vi "IB_RW_Convert_Path_to_Relative.vi"(8 "error in (no error)":errorcluster, 10 "commonPath":path, 11 "absolutePath":path) -> (0 "error out":errorcluster, 2 "relativeType":T1, 3 "newPath":path)   [LabVIEW 2020]
uses:
  <vilib>/AppBuilder/AB_Relative_Path_Type.ctl
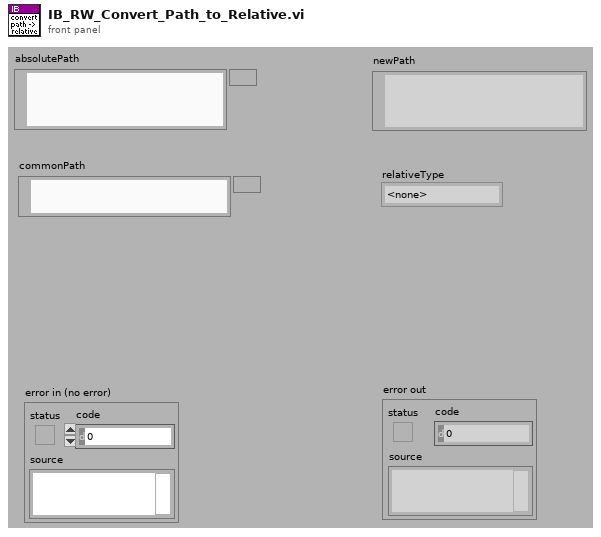
[diagram p1: front panel]
types:
  T1 = typedef "AB_Relative_Path_Type.ctl" = enum16{"<none>", "relativeToCommon", "relativeToAppDir", "relativeToProject"}
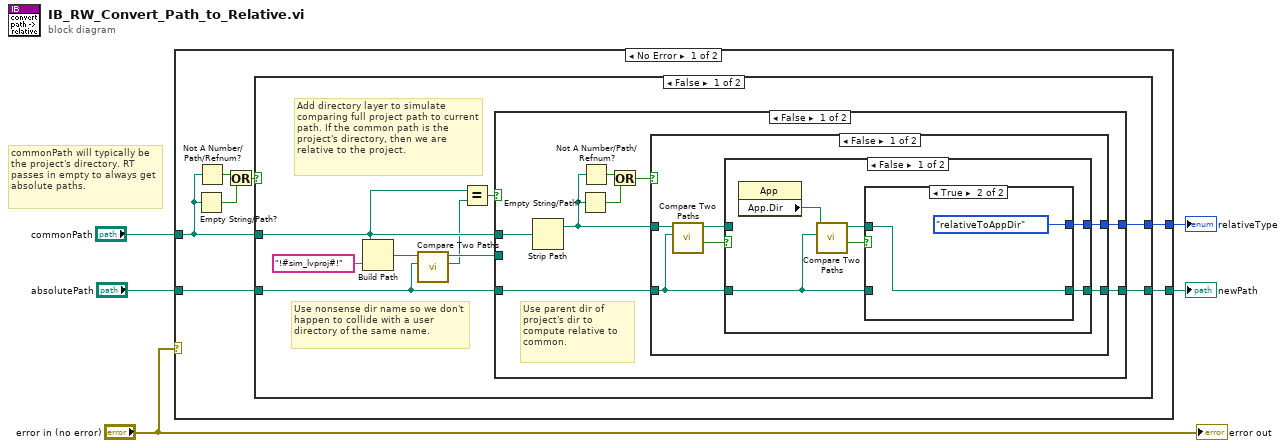
[diagram p0: block diagram]
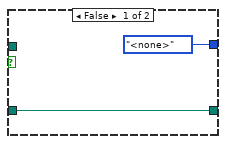
[diagram p2: hidden frame]
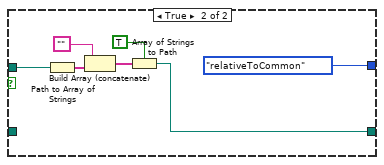
[diagram p3: hidden frame]
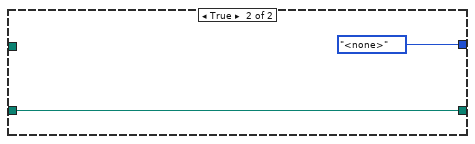
[diagram p4: hidden frame]
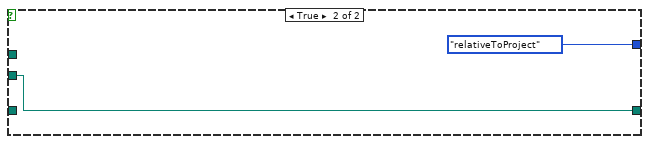
[diagram p5: hidden frame]
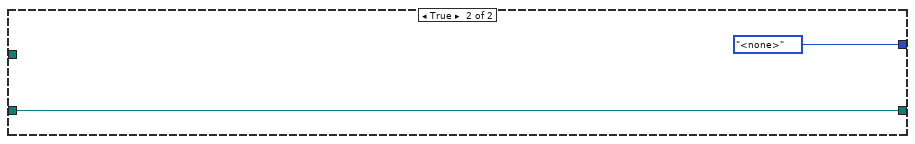
[diagram p6: hidden frame]
diagram:
  # "commonPath will typically be the project's directory. RT passes in empty to always get absolute paths."
  n1 = case shown="No Error" "error in (no error)" {
    tunnel: "commonPath" -> [w7 _]
    tunnel: "absolutePath" -> [w12 w59]
    tunnel: [w11 w59] -> w3
    tunnel: [w10 _] -> w2
    frame No Error {
      n2 = Empty String/Path?(string/path=w7) -> (empty?=w9:bool)
      n3 = Not A Number/Path/Refnum?(number/path/refnum=w7) -> (NaN/Path/Refnum?=w8:bool)
      n4 = Or(x=w8, y=w9) -> (x .or. y?=w6:bool)
      n5 = case shown="False" w6 {
        tunnel: w12 -> [w16 w58]
        tunnel: [w21 w58] -> w11
        tunnel: [w20 AB_Relative_Path_Type."<none>" ("relativeType")] -> w10
        tunnel: w7 -> [w15 _]
        frame False {
          # "Use nonsense dir name so we don't happen to collide with a user directory of the same name."
          # "Add directory layer to simulate comparing full project path to current path. If the common path is the project's directory, then we are relative to the project."
          n6 = Build Path(base path=w15, name or relative path="!#sim_lvproj#!") -> (appended path=w17:path)
          n7 = call <vilib>:"Compare Two Paths.vi"("Path 2"=w16, "Path 1"=w17) -> ("Common Path"=w14:path, "Relative Path from 1 to 2"=w18:path)  [unwired: 6 in, 2 out]
          n8 = Equal?(x=w15, y=w14) -> (x = y?=w13:bool)
          n9 = case shown="False" w13 {
            tunnel: [w29 w56] -> w21
            tunnel: [w28 AB_Relative_Path_Type."relativeToProject" ("relativeType")] -> w20
            tunnel: w15 -> [w23 _]
            tunnel: w16 -> [w22 _]
            tunnel: w18 -> [_ w56]
            frame False {
              # "Use parent dir of project's dir to compute relative to common."
              n10 = Strip Path(path=w23) -> (stripped path=w27:path)  [unwired: 1 out]
              n11 = Empty String/Path?(string/path=w27) -> (empty?=w25:bool)
              n12 = Not A Number/Path/Refnum?(number/path/refnum=w27) -> (NaN/Path/Refnum?=w26:bool)
              n13 = Or(x=w26, y=w25) -> (x .or. y?=w24:bool)
              n14 = case shown="False" w24 {
                tunnel: w22 -> [w34 w54]
                tunnel: [w33 w54] -> w29
                tunnel: [w32 AB_Relative_Path_Type."<none>" ("relativeType")] -> w28
                tunnel: w27 -> [w30 _]
                frame False {
                  n15 = call <vilib>:"Compare Two Paths.vi"("Path 2"=w34, "Path 1"=w30) -> ("Path 2 Relative to Path 1?"=w35:bool, "Relative Path from 1 to 2"=w31:path)  [unwired: 6 in, 2 out]
                  n16 = case shown="False" w35 {
                    tunnel: w34 -> [w38 _]
                    tunnel: [w39 w46] -> w33
                    tunnel: [w36 AB_Relative_Path_Type."relativeToCommon" ("relativeType")] -> w32
                    tunnel: w31 -> [_ w51]
                    frame False {
                      n17 = property class="App"() -> ("App.Dir"=w41:path)  [unwired: 2 in, 2 out]
                      n18 = call <vilib>:"Compare Two Paths.vi"("Path 2"=w38, "Path 1"=w41) -> ("Path 2 Relative to Path 1?"=w40:bool, "Relative Path from 1 to 2"=w37:path)  [unwired: 6 in, 2 out]
                      n19 = case shown="True" w40 {
                        tunnel: [w43 w45] -> w39
                        tunnel: w38 -> [w43 _]
                        tunnel: w37 -> [_ w45]
                        tunnel: [AB_Relative_Path_Type."<none>" ("relativeType") AB_Relative_Path_Type."relativeToAppDir" ("relativeType")] -> w36
                        frame False {
                        }
                        frame True {
                        }
                      }
                    }
                    frame True {
                      n20 = Path to Array of Strings(0:w51) -> (2:w50:string[])  [unwired: 1 out]
                      n21 = Build Array (concatenate)("", w50) -> (w48:string[])
                      n22 = Array of Strings to Path(0:w48, 1:TRUE ("relative")) -> (2:w46:path)
                    }
                  }
                }
                frame True {
                }
              }
            }
            frame True {
            }
          }
        }
        frame True {
        }
      }
    }
    frame Error {
    }
  }
  "newPath" <- w3
  "relativeType" <- w2
  "error out" <- "error in (no error)"
